vi "HelpOn.vi"(8 "Error In":errorcluster, 11 "reference in":refnum<class "Clippy.lvclass">) -> (0 "Error Out":errorcluster, 3 "reference out":refnum<class "Clippy.lvclass">)   [LabVIEW 2020, in "Clippy.lvclass"]
uses:
  Clippy.lvclass
  AnimationTypes.ctl
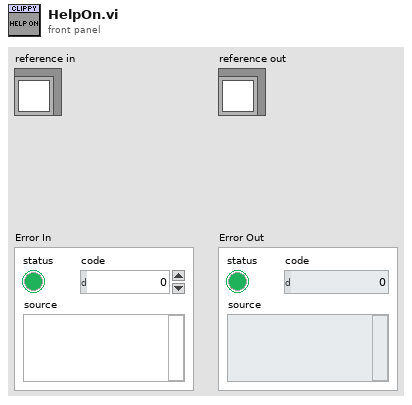
[diagram p1: front panel]
types:
  T1 = typedef "Clippy.lvclass/AnimationTypes.ctl" = enum16{"Congratulate", "LookRight", "SendMail", "Thinking", "Explain", "IdleRopePile", "IdleAtom", "Print", "Hide", "GetAttention", "Save", "GetTechy", "GestureUp", "Idle1_1", "Processing", "Alert", "LookUpRight", "IdleSideToSide", "GoodBye", "LookLeft", "IdleHeadScratch", "LookUpLeft", "CheckingSomething", "Hearing_1", "GetWizardy", "IdleFingerTap", "GestureLeft", "Wave", "GestureRight", "Writing", "IdleSnooze", "LookDownRight", "GetArtsy", "Show", "LookDown", "Searching", "EmptyTrash", "Greeting", "LookUp", "GestureDown", "RestPose", "IdleEyeBrowRaise", "LookDownLeft"}
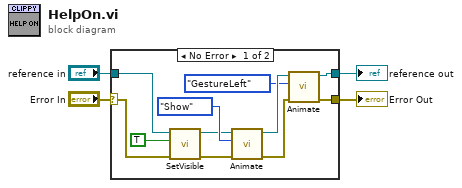
[diagram p0: block diagram]
diagram:
  n1 = case shown="No Error" "Error In" {
    selector: "Error In" -> [w9 w17]
    tunnel: [w11 w17] -> w3
    tunnel: [w10 w16] -> w1
    tunnel: "reference in" -> [w6 w16]
    frame No Error {
      n2 = call "SetVisible.vi"("Error In"=w9, "Visible"=TRUE, "reference in"=w6) -> ("Error Out"=w8:errorcluster, "reference out"=w7:refnum<class "Clippy.lvclass">)  [unwired: 7 in]
      n3 = call-dynamic "Animate.vi"("Error In"=w8, "Animation"=AnimationTypes."Show", "reference in"=w7) -> ("Error Out"=w14:errorcluster, "reference out"=w13:refnum<class "Clippy.lvclass">)  [unwired: 7 in]
      n4 = call-dynamic "Animate.vi"("Error In"=w14, "Animation"=AnimationTypes."GestureLeft", "reference in"=w13) -> ("Error Out"=w11:errorcluster, "reference out"=w10:refnum<class "Clippy.lvclass">)  [unwired: 7 in]
    }
    frame Error {
    }
  }
  "Error Out" <- w3
  "reference out" <- w1
